vi "Filter Graves.vi"(8 "Error In":errorcluster) -> (0 "Error Out":errorcluster)   [LabVIEW 2018, in "Tests.lvlib" / "Toolkit.lvlib" / "Integration.lvlib"]
uses:
  Integration.lvlib
  <vilib>/Utility/traverseref.llb/TRef TravTarget.ctl
  <vilib>/addons/_JKI Toolkits/Caraya/classes/Test/Test.lvclass
  <vilib>/addons/_JKI Toolkits/Caraya/classes/Assert/Assert.lvclass
  <vilib>/Utility/traverseref.llb/VI Scripting - Traverse.lvlib
  src/Toolkit/Toolkit.lvlib
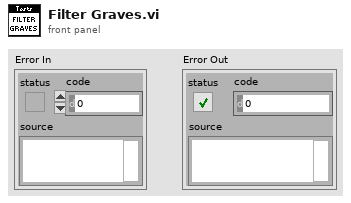
[diagram p1: front panel]
types:
  T1 = typedef "TRef TravTarget.ctl" = enum16{"FP", "BD", "Other"}
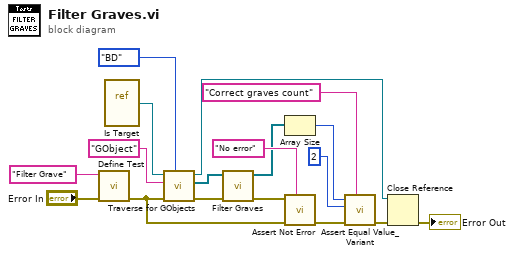
[diagram p0: block diagram]
diagram:
  n1 = call <vilib>:"Define Test.vi"("error in (no error)"="Error In", "Label (VI Title)"="Filter Grave") -> ("error out"=w10:errorcluster)  [unwired: 9 in]
  n2 = vi-ref "Is Target.vi"() -> (w9:refnum<vi>)
  n3 = call <vilib>:"Traverse for GObjects.vi"("Traverse Target"=TRef_TravTarget."BD", "error in (no error)"=w10, "Class Name"="GObject", "VI Refnum"=w9) -> ("error out"=w3:errorcluster, "References"=w4:refnum<vi>[], "dup VI Refnum"=w6:refnum<vi>)  [unwired: 4 in, 1 out]
  n4 = call "Filter Graves.vi"("Error In"=w3, "GObjects"=w4) -> ("Error Out"=w2:errorcluster, "Graves"=w1:refnum<vi>[])  [unwired: 8 in]
  n5 = Array Size(array=w1) -> (size(s)=w12:i32)
  n6 = call <vilib>:"Assert Not Error.vi"("Label"="No error", "error in (no error)"=w10, "Not Error?"=w2) -> ("error out"=w16:errorcluster)  [unwired: 8 in]
  n7 = call <vilib>:"Assert Equal Value_Variant.vi"("Label"="Correct graves count", "error in (no error)"=w16, "Y"=2 ("size(s)"), "X"=w12) -> ("error out"=w13:errorcluster)  [unwired: 7 in]
  n8 = Close Reference(reference=w6, error in (no error)=w13) -> (error out=→"Error Out":errorcluster)
